vi "ModbusRead.vi"() -> (0 "error out":errorcluster, 1 "register values":u16[](array[numeric]))   [LabVIEW 2024]
uses:
  <vilib>/Modbus/master/Create Master Instance (TCP).vi
  <vilib>/Modbus/master/Modbus Master.lvclass
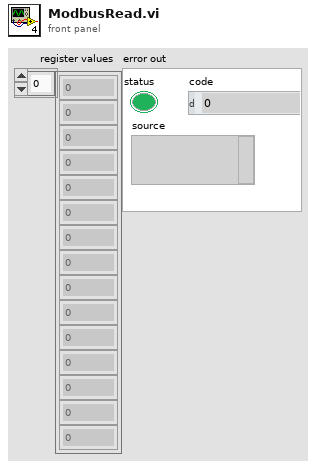
[diagram p1: front panel]
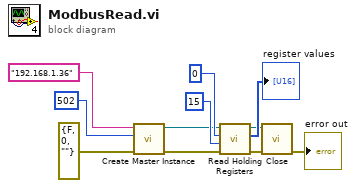
[diagram p0: block diagram]
diagram:
  n1 = call-poly <vilib>:"Create Master Instance.vi"("error in (no error)"=errorcluster {"status"=FALSE, "code"=0, "source"=""}, "port (502)"=u16 502, "address"="192.168.1.36") -> ("error out"=w4:errorcluster, "TCP master instance"=w5:refnum<class "Modbus Master.lvclass">)  [unwired: 7 in]
  n2 = call-dynamic "Read Holding Registers.vi"("error in (no error)"=w4, "number of holding registers"=u16 15, "starting address"=u16 0, "Modbus master in"=w5) -> ("error out"=w1:errorcluster, "register values"=→"register values":u16[], "Modbus master out"=w2:refnum<class "Modbus Master.lvclass">)  [unwired: 5 in]
  n3 = call-dynamic "Close.vi"("error in (no error)"=w1, "Modbus master in"=w2) -> ("error out"=→"error out":errorcluster)  [unwired: 9 in]
